vi "Pasco Dead Band.vi"(8 "lower limit":dbl, 9 "PWM Power":dbl, 10 "upper limit":dbl) -> (0 "Integral Reset":bool, 3 "PWM Power":dbl)   [LabVIEW 2014]
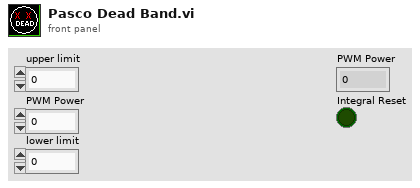
[diagram p1: front panel]
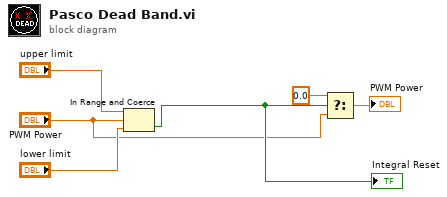
[diagram p0: block diagram]
diagram:
  n1 = In Range and Coerce(upper limit="upper limit", x="PWM Power", lower limit="lower limit") -> (In Range?=w4:bool)  [unwired: 1 out]
  "Integral Reset" <- w4
  n2 = Select(t=0.0, s=w4, f="PWM Power") -> (s? t:f=→"PWM Power":dbl)
